vi "ShooterStop.vi"(9 "Run":bool, 11 "Button":bool) -> (3 "StopShooter?":bool)   [LabVIEW 2015]
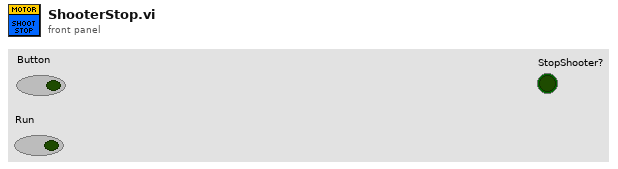
[diagram p1: front panel]
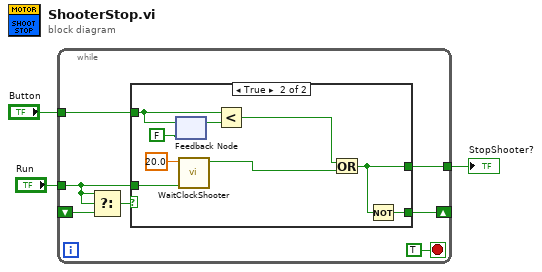
[diagram p0: block diagram]
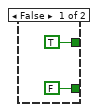
[diagram p2: hidden frame]
diagram:
  n1 = while {
    tunnel: "Run" -> [w7]
    tunnel: "Button" -> [w10]
    shift-right: [w4] -> _
    shift-left: _ -> [w8]
    tunnel: [w5] -> w1
    stop <- TRUE stop-if-true
    n2 = Select(t=w7, s=w7, f=w8) -> (s? t:f=w6:bool)
    n3 = case shown="True" w6 {
      tunnel: w10 -> [_ w21]
      tunnel: w7 -> [_ w17]
      tunnel: [TRUE w15] -> w5
      tunnel: [FALSE w14] -> w4
      frame False {
      }
      frame True {
        n4 = feedback #1(FALSE ("Button")) -> (w20:bool)
        n5 = feedback-in #1(w21) -> ()
        n6 = call "WaitClockShooter.vi"("First Time?"=w17, "Target Time"=20.0) -> ("Completed"=w18:bool)  [unwired: 9 in]
        n7 = Less?(x=w21, y=w20) -> (x < y?=w13:bool)
        n8 = Or(x=w13, y=w18) -> (x .or. y?=w15:bool)
        n9 = Not(x=w15) -> (.not. x?=w14:bool)
      }
    }
  }
  "StopShooter?" <- w1
